vi "test.vi"(5 "stop":bool) -> (2 "Array":string[](array[string]), 3 "Waveform Chart":dynamicdata(graph))   [LabVIEW 2022 SP3]
uses:
  <vilib>/Platform/TimedLoop/XDataNode/timing_clust.ctl
  <vilib>/Platform/TimedLoop/XDataNode/nitl_modes.ctl
  <vilib>/Platform/TimedLoop/XDataNode/wakeup.ctl
  <vilib>/Utility/file.llb/Write Delimited Spreadsheet (string).vi
  <vilib>/platform/TimedLoop/XDataNode/XDataNode.xnode
  <vilib>/Instr/_visa.llb/VISA Configure Serial Port (Instr).vi
  <vilib>/Platform/TimedLoop/XDataNode/XDNodeRunTimeDep.lvlib
panel:
  out "Table Control":string[][](table)
  in  "Desired Temp":dbl(knob)=25.0 step=0.1 scale=15.0..30.0 scale format="%#_2g"
  out "Room Temp":dbl(slide) scale=10.0..30.0
  out "appended array 2":string[](array[string])
  out "read buffer":string
  in  "file path (dialog if empty)":path=path "C:/Users/celin/Documents/Alexandre Escola/Universidade/FEUP - Faculdade de Engenharia do Porto/1º Semestre/ASM - Aplicações de Sistemas Mecatrónicos/Arduino+LabView/test.xls"
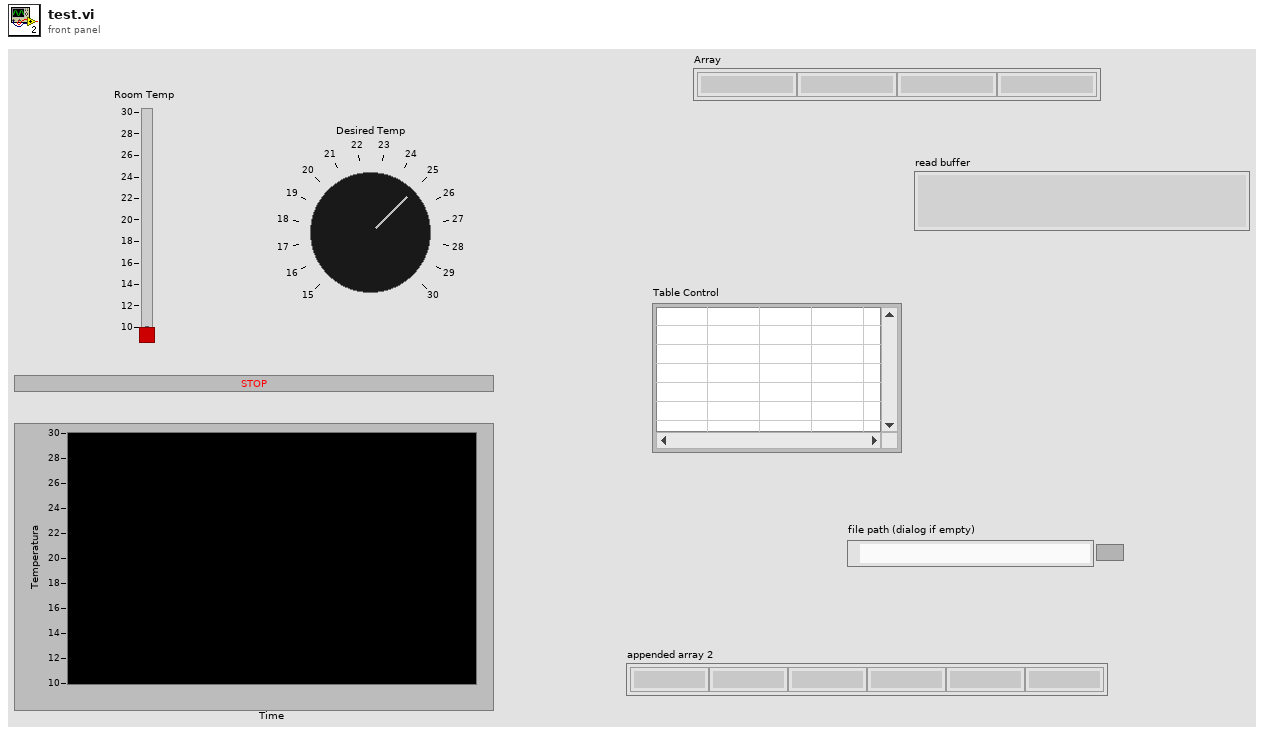
[diagram p1: front panel]
types:
  T1 = typedef "XDNodeRunTimeDep.lvlib/timing_clust.ctl" = cluster{"Expected End [f-1]":u64, "Actual End [f-1]":u64, "Finished Late? [f-1]":bool, "Expected End [i-1]":u64, "Actual End [i-1]":u64, "Finished Late? [i-1]":bool, "Expected Start [i]":u64, "Actual Start [i]":u64, "Expected Start [f]":u64, "Actual Start [f]":u64, "Source Name":string, "Structure Name":string, "Period":i64, "Deadline":i64, "Offset":i64, "Start":i64, "Priority":i32, "Timeout":i32, "Mode":T2, "Wakeup Reason":T3, "Error":errorcluster, "Source Type":string, "Secondary Source Type":string, "Global End Time":u64, "Global Start Time":u64, "Frame Duration":u64, "Iteration Duration":u64, "Assigned CPU":i32, "I/O Scan Engine Mode":u32}
  T2 = typedef "XDNodeRunTimeDep.lvlib/nitl_modes.ctl" = enum32{"No Change", "Process missed periods, maintain original phase", "Discard missed periods, maintain original phase", "Process missed periods, ignore original phase", "Discard missed periods, ignore original phase"}
  T3 = typedef "XDNodeRunTimeDep.lvlib/wakeup.ctl" = enum32{"Normal", "Aborted", "Asynchronous wakeup", "Timing source error", "Timed loop error", "Timeout"}
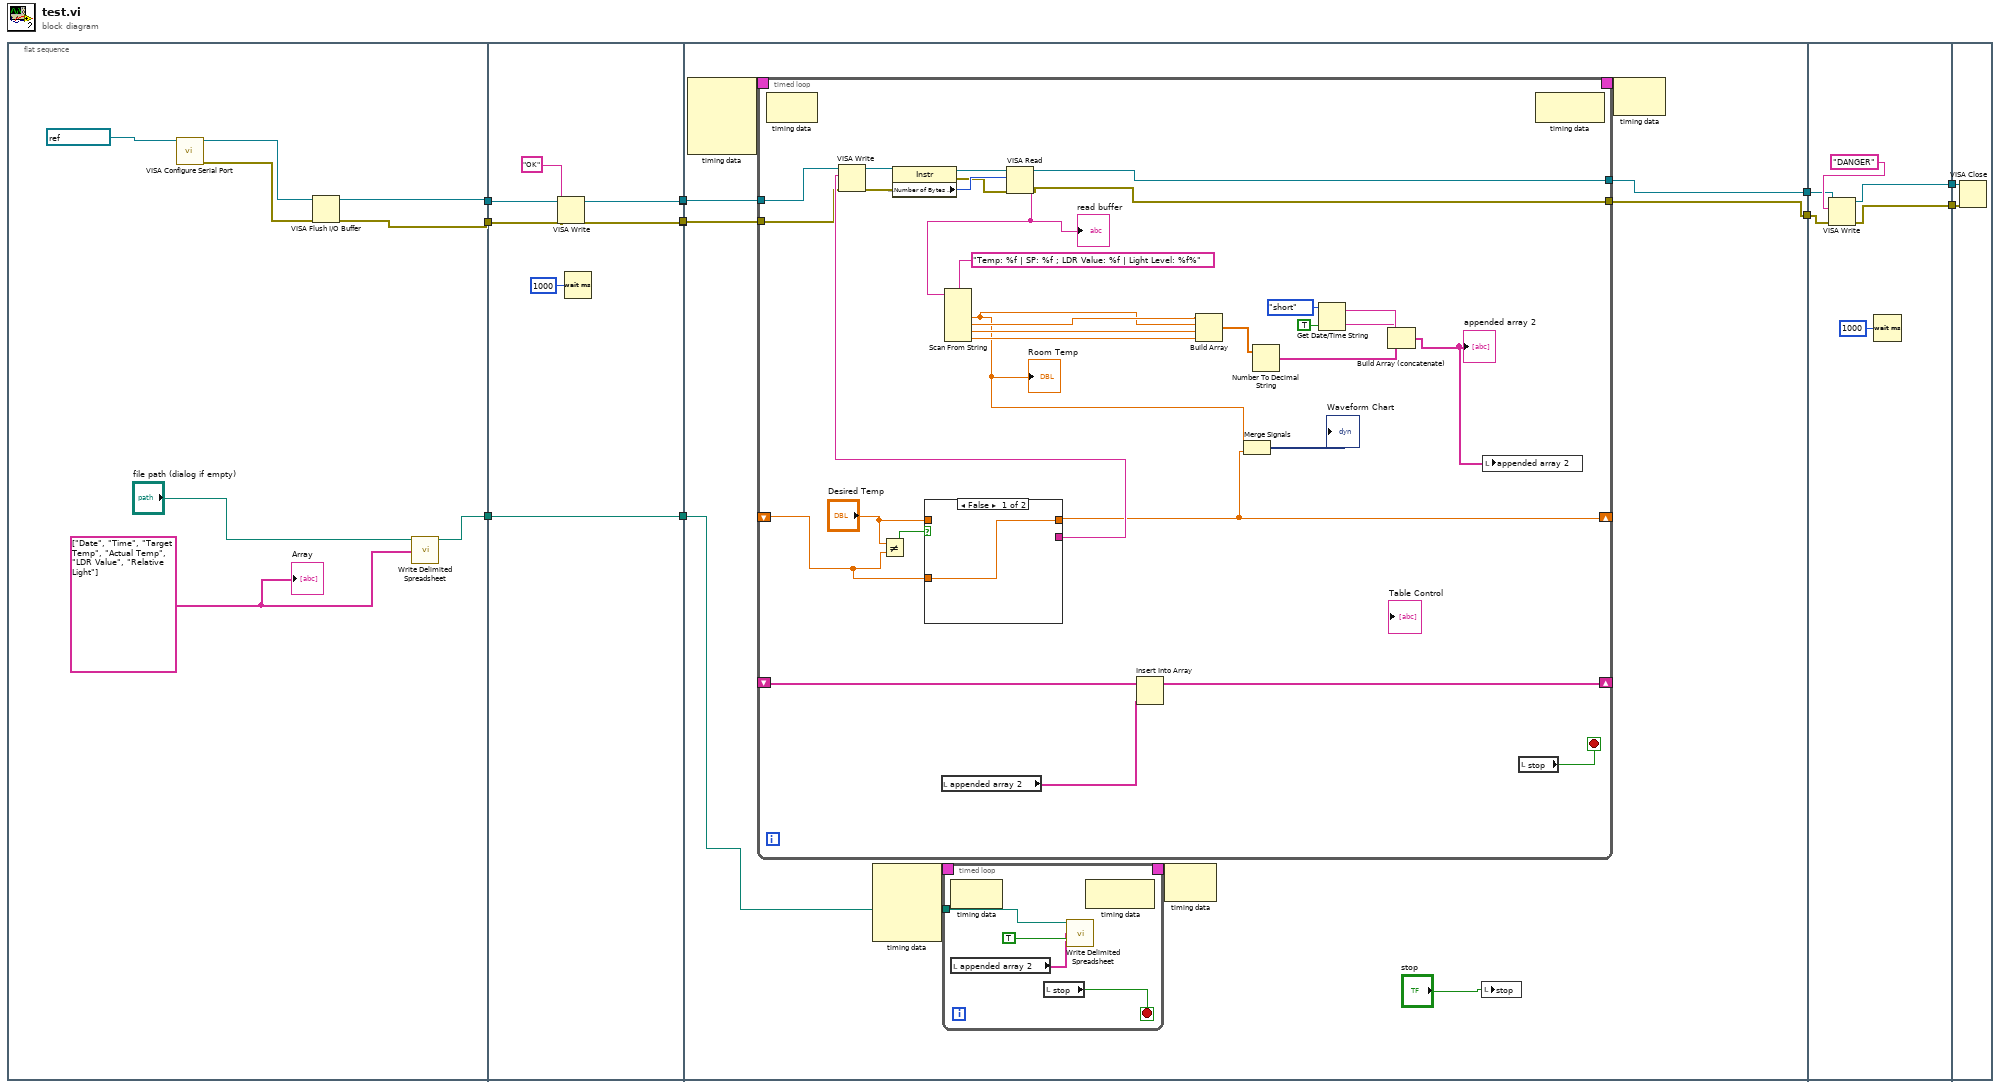
[diagram p0: block diagram]
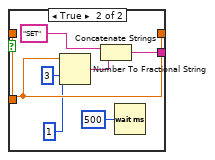
[diagram p2: hidden frame]
diagram:
  n1 = flat-sequence {
    tunnel: [w14] -> w8
    tunnel: [w15] -> w6
    tunnel: [w19] -> w4
    tunnel: w8 -> [w27]
    tunnel: [w27] -> w7
    tunnel: w6 -> [w26]
    tunnel: [w26] -> w5
    tunnel: w4 -> [w25]
    tunnel: [w25] -> w3
    tunnel: [w24] -> w2
    tunnel: [w23] -> w1
    tunnel: w7 -> [_]
    tunnel: w5 -> [_]
    tunnel: w3 -> [w31]
    tunnel: [w37] -> w12
    tunnel: [w36] -> w11
    tunnel: w2 -> [w30]
    tunnel: w1 -> [w29]
    tunnel: w12 -> [w95]
    tunnel: w11 -> [w93]
    tunnel: [w92] -> w10
    tunnel: [w91] -> w9
    tunnel: w10 -> [w97]
    tunnel: w9 -> [w96]
    frame #0 {
      w18 = string[] ["Date", "Time", "Target Temp", "Actual Temp", "LDR Value", "Relative Light"]
      n2 = call-poly "VISA Configure Serial Port"("VISA resource name"=refnum<visa-resource-name> "COM3-1" ("Port Name")) -> ("VISA resource name out"=w17:refnum<visa-resource-name>, "error out"=w16:errorcluster)  [unwired: 13 in]
      n3 = VISA Flush I/O Buffer(VISA resource name=w17, error in (no error)=w16) -> (VISA resource name out=w14:refnum<visa-resource-name>, error out=w15:errorcluster)  [unwired: 1 in]
      n4 = call-poly <vilib>:"Write Delimited Spreadsheet.vi"("file path (dialog if empty)"="file path (dialog if empty)", "1D data"=w18) -> ("new file path (Not A Path if cancelled)"=w19:path)  [unwired: 12 in, 1 out]
      "Array" <- w18
    }
    frame #1 {
      n5 = VISA Write(VISA resource name=w27, write buffer="OK", error in (no error)=w26) -> (VISA resource name out=w23:refnum<visa-resource-name>, error out=w24:errorcluster)  [unwired: 1 out]
      n6 = Wait (ms)(milliseconds to wait=u32 1000) -> ()  [unwired: 1 out]
    }
    frame #2 {
      n7 = node-c288() -> (w35:T1)  [unwired: 4 in]
      n8 = timed-loop {
        tunnel: [w77] -> w36
        tunnel: [w76] -> w37
        shift-right: [w56] -> _
        shift-left: _ -> [w57]
        timing: w35 -> [_]
        timing-out: [_] -> w34
        tunnel: w30 -> [w52]
        tunnel: w29 -> [w51]
        shift-right: [w46] -> _
        shift-left: _ -> [w49]
        stop <- w50 stop-if-true
        n9 = node-c288() -> ()  [unwired: 1 in, 1 out]
        n10 = Not Equal?(x="Desired Temp", y=w57) -> (x != y?=w59:bool)
        n11 = case shown="False" w59 {
          tunnel: [w80 w85] -> w56
          tunnel: "Desired Temp" -> [_ w85]
          tunnel: [_ w83] -> w63
          tunnel: w57 -> [w80 _]
          frame False {
          }
          frame True {
            n12 = Number To Fractional String(number=w85, width (-)=i16 3, precision (6)=i16 1 ("width (-)")) -> (F-format string=w86:string)  [unwired: 1 in]
            n13 = Concatenate Strings("SET", w86) -> (w83:string)
            n14 = Wait (ms)(milliseconds to wait=u32 500) -> ()  [unwired: 1 out]
          }
        }
        n15 = VISA Write(VISA resource name=w51, write buffer=w63, error in (no error)=w52) -> (VISA resource name out=w61:refnum<visa-resource-name>, error out=w60:errorcluster)  [unwired: 1 out]
        n16 = property class="Instr"(reference=w61, error in=w60) -> (reference out=w75:refnum<visa-resource-name>, error out=w73:errorcluster, "Serial Settings:Number of Bytes at Serial Port"=w74:u32)
        n17 = local read "appended array 2"() -> (w47:string[])
        n18 = VISA Read(VISA resource name=w75, byte count=w74, error in (no error)=w73) -> (VISA resource name out=w77:refnum<visa-resource-name>, read buffer=w72:string, error out=w76:errorcluster)  [unwired: 1 out]
        "read buffer" <- w72
        n19 = Scan From String(format string="Temp: %f | SP: %f ; LDR Value: %f | Light Level: %f%", input string=w72) -> (output 1=w54:dbl, output 2=w64:dbl, output 3=w70:dbl, output 4=w69:dbl)  [unwired: 6 in, 3 out]
        "Room Temp" <- w54
        n20 = Insert Into Array(array=w49, new element=w47) -> (w46:string[])  [unwired: 1 in]
        n21 = Build Array(w64, w54, w70, w69) -> (w53:dbl[])
        n22 = Merge Signals(w54, w56) -> (→"Waveform Chart":dynamicdata)
        n23 = Number To Decimal String(number=w53) -> (decimal integer string=w67:string[])  [unwired: 1 in]
        n24 = Get Date/Time String(date format (0)=enum16{"short", "long", "abbreviated"}."short", want seconds? (F)=TRUE) -> (date string=w66:string, time string=w65:string)  [unwired: 1 in]
        n25 = Build Array (concatenate)(w66, w65, w67) -> (w48:string[])
        "appended array 2" <- w48
        n26 = local write "appended array 2"(w48) -> ()
        n27 = local read "stop"() -> (w50:bool)
        n28 = node-c288() -> ()  [unwired: 1 in, 1 out]
      }
      n29 = node-c288() -> (w33:T1)  [unwired: 4 in]
      n30 = timed-loop {
        timing: w33 -> [_]
        timing-out: [_] -> w32
        tunnel: w31 -> [w41]
        stop <- w39 stop-if-true
        n31 = node-c288() -> ()  [unwired: 1 in, 1 out]
        n32 = local read "appended array 2"() -> (w38:string[])
        n33 = local read "stop"() -> (w39:bool)
        n34 = call-poly <vilib>:"Write Delimited Spreadsheet.vi"("file path (dialog if empty)"=w41, "1D data"=w38, "append to file? (new file:F)"=TRUE) -> ()  [unwired: 11 in, 2 out]
        n35 = node-c288() -> ()  [unwired: 1 in, 1 out]
      }
      n36 = node-c288(w32) -> ()  [unwired: 1 out]
      n37 = local write "stop"("stop") -> ()
      n38 = node-c288(w34) -> ()  [unwired: 1 out]
    }
    frame #3 {
      n39 = VISA Write(VISA resource name=w93, write buffer="DANGER", error in (no error)=w95) -> (VISA resource name out=w91:refnum<visa-resource-name>, error out=w92:errorcluster)  [unwired: 1 out]
      n40 = Wait (ms)(milliseconds to wait=u32 1000) -> ()  [unwired: 1 out]
    }
    frame #4 {
      n41 = VISA Close(VISA resource name=w96, error in (no error)=w97) -> ()  [unwired: 1 out]
    }
  }
